vi "AccumulatingAnswers.vi"(8 "wrong":i32, 9 "right":i32, 10 "Label":sgl format="%#_13g", 11 "Output":sgl[](array[numeric]) format="%#_13g") -> (0 "wrong":i32, 3 "right":i32)   [LabVIEW 2020]
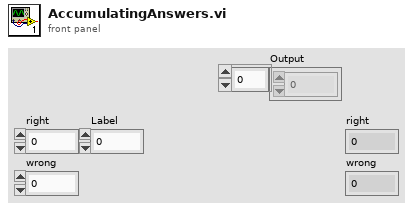
[diagram p1: front panel]
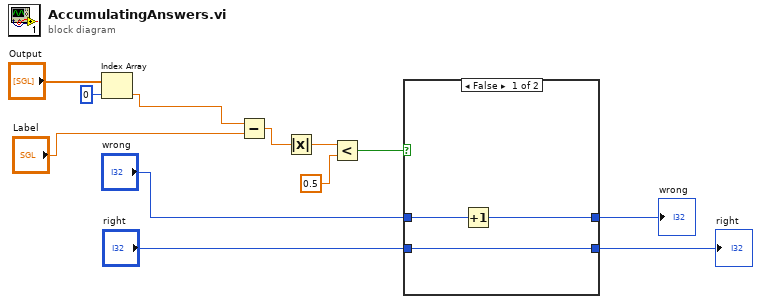
[diagram p0: block diagram]
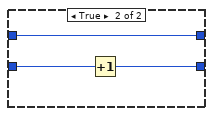
[diagram p2: hidden frame]
diagram:
  n1 = Index Array(array="Output", index=0) -> (element=w4:sgl)
  n2 = Subtract(x=w4, y="Label") -> (x-y=w2:sgl)
  n3 = Absolute Value(x=w2) -> (abs(x)=w3:sgl)
  n4 = Less?(x=w3, y=sgl 0.5) -> (x < y?=w1:bool)
  n5 = case shown="False" w1 {
    tunnel: "right" -> [w13 w18]
    tunnel: [w13 w17] -> w10
    tunnel: "wrong" -> [w15 w16]
    tunnel: [w14 w16] -> w8
    frame False {
      n6 = Increment(x=w15) -> (x+1=w14:i32)
    }
    frame True {
      n7 = Increment(x=w18) -> (x+1=w17:i32)
    }
  }
  "right" <- w10
  "wrong" <- w8
